vi "test_WFGenerate01DC.vi"() -> ()   [LabVIEW 2009]
panel:
  out "Waveform Out":waveform(dbl)
  in  "Param 3":dbl
  in  "Param 2":dbl
  in  "Param 1":dbl
  in  "Param 0":dbl
  in  "Waveform Properties":T1 {"Ramp (s)" min=0.0; "Fs (Hz)" min=0.0}
  out "Waveform Graph":waveform(dbl)(graph)
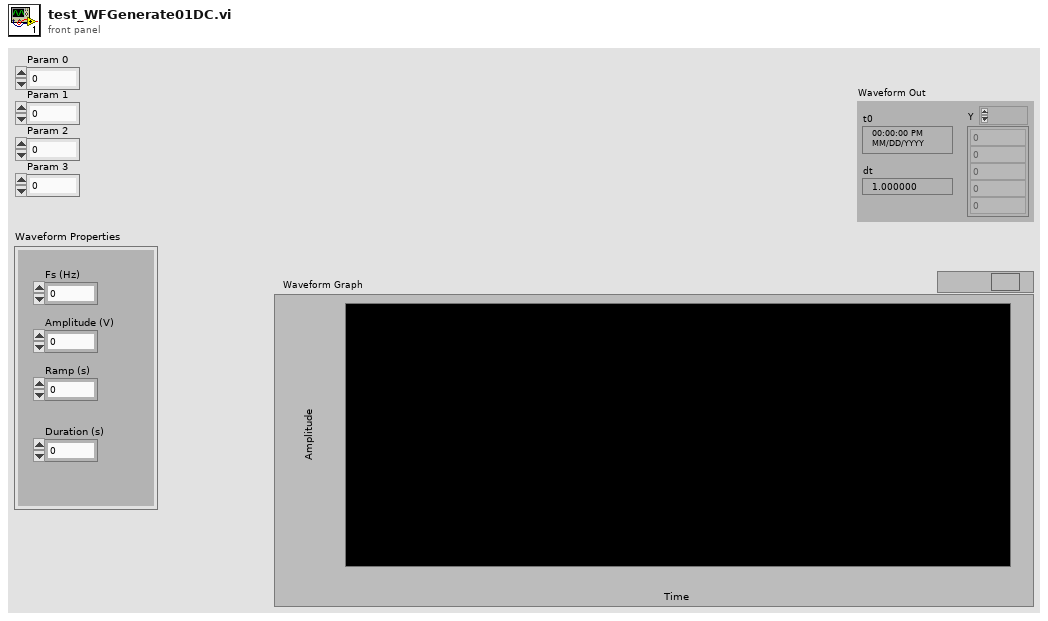
[diagram p1: front panel]
types:
  T1 = cluster{"Fs (Hz)":dbl, "Amplitude (V)":dbl, "Ramp (s)":dbl, "Duration (s)":dbl}
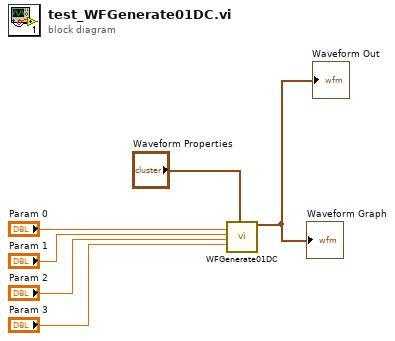
[diagram p0: block diagram]
diagram:
  n1 = call "WFGenerate01DC.vi"("Param 0"="Param 0", "Param 1"="Param 1", "Param 2"="Param 2", "Param 3"="Param 3", "Waveform Properties"="Waveform Properties") -> ("Waveform Out"=→"Waveform Graph" →"Waveform Out":waveform(dbl))  [unwired: 13 in, 1 out]
